vi "Threshold Exceeded.vi"() -> ()   [LabVIEW 2019]
uses:
  <vilib>/DAQmx/read.llb/DAQmx Read (Analog DBL 1Chan 1Samp).vi
  <vilib>/DAQmx/create/channels.llb/DAQmx Create Channel (AI-Temperature-Thermocouple).vi
  <vilib>/DAQmx/configure/timing.llb/DAQmx Timing (Sample Clock).vi
  <vilib>/DAQmx/miscellaneous.llb/DAQmx Fill In Error Info.vi
panel:
  out "Threshold Ever Exceeded?":bool
  out "Threshold Currently Exceeded?":bool
  in  "Max Threshold (deg C)":dbl
  in  "Stop":bool
  out "Temperature Chart":dbl(graph)
  in  "Thermocouple Channel":tag="PCI-6221/ai0"
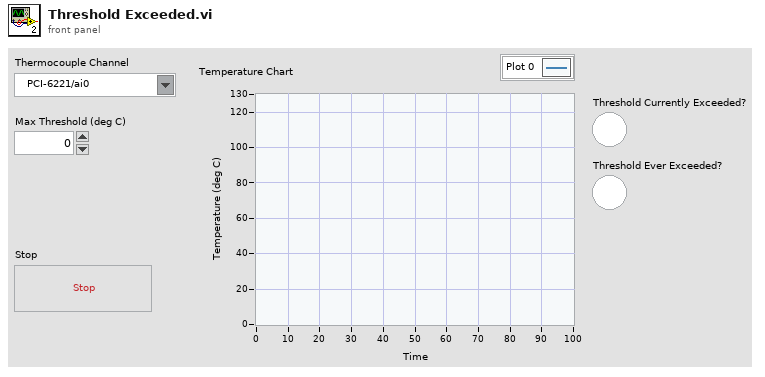
[diagram p1: front panel]
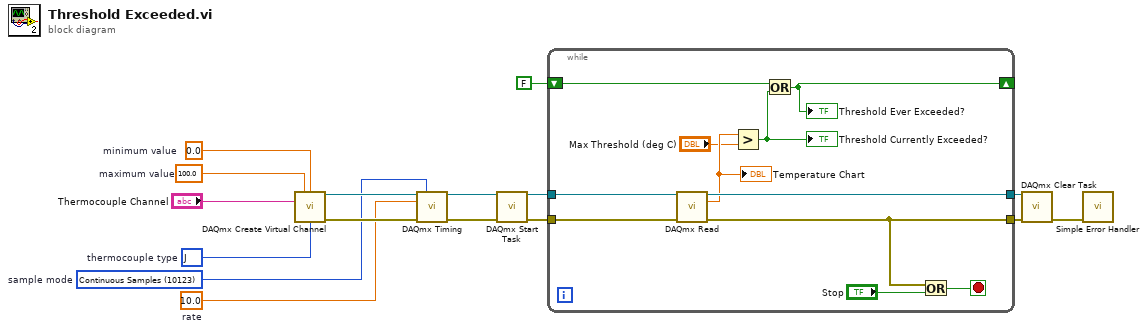
[diagram p0: block diagram]
diagram:
  w10 = 10072 items=["J"=10072, "K"=10073, "N"=10077, "R"=10082, "S"=10085, "T"=10086, "B"=10047, "E"=10055]  # thermocouple type
  w11 = 0.0  # minimum value
  w12 = 100.0  # maximum value
  w13 = 10.0  # rate
  w14 = 10123 items=["Finite Samples"=10178, "Continuous Samples"=10123, "Hardware Timed Single Point"=12522]  # sample mode
  n1 = call-poly <vilib>:"DAQmx Create Virtual Channel.vi"("maximum value"=w12, "minimum value"=w11, "physical channels"="Thermocouple Channel", "thermocouple type"=w10) -> ("task out"=w16:refnum<k21>, "error out"=w15:errorcluster)  [unwired: 10 in]
  n2 = call-poly <vilib>:"DAQmx Timing.vi"("task/channels in"=w16, "sample mode"=w14, "rate"=w13, "error in"=w15) -> ("task out"=w8:refnum<k21>, "error out"=w7:errorcluster)  [unwired: 10 in]
  n3 = call <vilib>:"DAQmx Start Task.vi"("task/channels in"=w8, "error in"=w7) -> ("task out"=w6:refnum<k21>, "error out"=w5:errorcluster)  [unwired: 12 in]
  n4 = while {
    tunnel: w6 -> [w27]
    tunnel: [w25] -> w4
    tunnel: w5 -> [w26]
    tunnel: [w24] -> w3
    shift-right: [w17] -> _
    shift-left: FALSE -> [w19]
    stop <- w23 stop-if-true
    n5 = call-poly <vilib>:"DAQmx Read.vi"("task/channels in"=w27, "error in"=w26) -> ("task out"=w25:refnum<k21>, "data"=w21:dbl, "error out"=w24:errorcluster)  [unwired: 11 in]
    "Temperature Chart" <- w21
    n6 = Greater?(x=w21, y="Max Threshold (deg C)") -> (0:w18:bool)
    "Threshold Currently Exceeded?" <- w18
    n7 = Or(x=w19, y=w18) -> (x .or. y?=w17:bool)
    "Threshold Ever Exceeded?" <- w17
    n8 = Or(x=w24, y="Stop") -> (x .or. y?=w23:bool)
  }
  n9 = call <vilib>:"DAQmx Clear Task.vi"("task in"=w4, "error in"=w3) -> ("error out"=w2:errorcluster)  [unwired: 13 in]
  n10 = call <vilib>:"Simple Error Handler.vi"("error in (no error)"=w2) -> ()  [unwired: 4 in, 5 out]
